vi "Launcher - Table.vi"(6 "Worker Alias":string="Table", 9 "Initialization Data":T1={"# Philosophers"=5} {"# Philosophers" min=5 max=500 step=1}, 11 "Table in":refnum<class "Table.lvclass">) -> ()   [LabVIEW 2021]
doc: "This VI launches the Head Worker of a Workers application."
uses:
  Workers/Table/Table.lvclass
  <vilib>/addons/_Workers/Debugger/Debug Client/Debug Client.lvlib
  Utility/Utility.lvlib
  Workers/Table/Initialization Data.ctl
panel:
  in  "# Philosophers":i32=5 min=5 max=500 step=1
  # "Overview:  https://en.wikipedia.org/wiki/Dining_philosophers_problem\n\nRequirements:  LabVIEW 2025 Q1   Workers SDK 5.0  by Scarfe Controls\n\n                              https://www.workersforlabview.com/\n\nExample Chapter 9.2 The Dining Philosopher Problem  https://www.state-machine.com/psicc2"
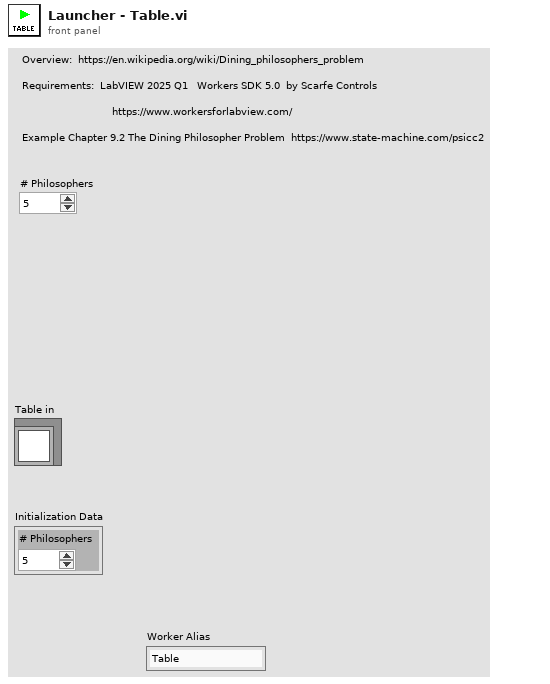
[diagram p1: front panel]
types:
  T1 = typedef "Table.lvclass/Initialization Data.ctl" = cluster{"# Philosophers":i32}
  T2 = enum32{"Invalid", "Standard", "Closed", "Hidden", "Minimized", "Maximized"}
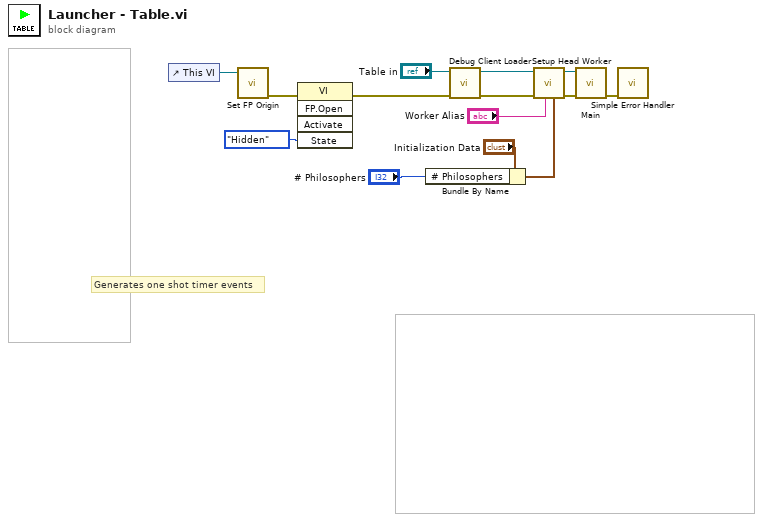
[diagram p0: block diagram]
diagram:
  # "Generates one shot timer events"
  n1 = control-ref of="This VI"() -> (w2:refnum<vi>)
  n2 = call "Set FP Origin.vi"("VI ref in"=w2) -> ("error out"=w10:errorcluster)  [unwired: 9 in, 1 out]
  n3 = invoke class="VI" method="FP.Open"(error in=w10, "State"=T2."Hidden") -> (error out=w11:errorcluster)  [unwired: 3 in, 4 out]
  n4 = Bundle By Name(cluster="Initialization Data", "# Philosophers"="# Philosophers") -> (w1:T1)
  n5 = call <vilib>:"Debug Client Loader.vi"("error in (no error)"=w11, "Worker_"="Table in") -> ("error out"=w12:errorcluster, "Worker_out"=w6:refnum<class "Table.lvclass">)  [unwired: 8 in]
  n6 = call-dynamic "Setup Head Worker.vi"("Initalization Data"=w1, "Worker Alias"="Worker Alias", "error in"=w12, "Worker_"=w6) -> ("error out"=w14:errorcluster, "Worker_out"=w9:refnum<class "Table.lvclass">)  [unwired: 6 in]
  n7 = call-dynamic "Main.vi"("error in"=w14, "Table in"=w9) -> ("error out"=w13:errorcluster)  [unwired: 8 in, 1 out]
  n8 = call <vilib>:"Simple Error Handler.vi"("error in (no error)"=w13) -> ()  [unwired: 4 in, 5 out]
